vi "JSON Add Indent.vi"(8 "error in (no error)":errorcluster, 10 "Indent Size (2)":u32=2, 11 "JSON String":string) -> (0 "error out":errorcluster, 3 "Indented JSON String":string)   [LabVIEW 2020, in "RxnRover.lvlib" / "File IO.lvlib" / "JSON Utilities.lvlib"]
doc: "Adds indentation to the JSON string provided. The string must already have newlines added for indentation to be useful."
uses:
  JSON Utilities.lvlib
  <vilib>/regexp/Match Regular Expression.xnode
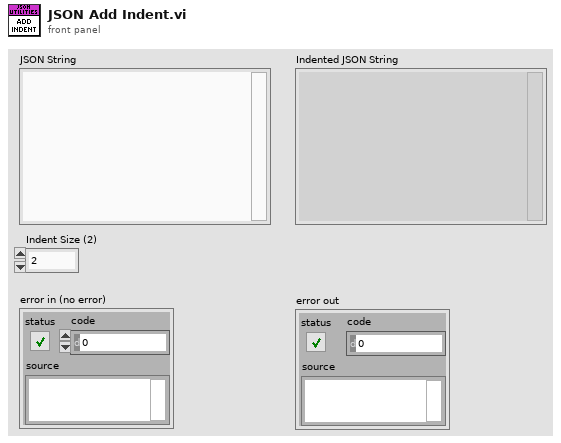
[diagram p1: front panel]
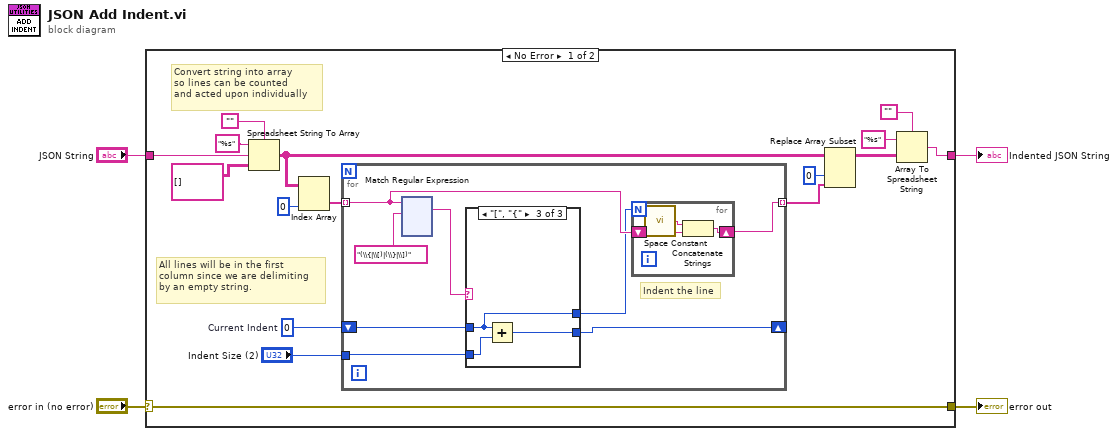
[diagram p0: block diagram]
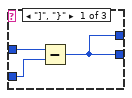
[diagram p2: hidden frame]
diagram:
  n1 = case shown="No Error" "error in (no error)" {
    selector: "error in (no error)" -> [w5 w154]
    tunnel: "JSON String" -> [w19 w153]
    tunnel: [w8 w153] -> w3
    tunnel: [w5 w154] -> w1
    frame No Error {
      w6 = 0  # Current Indent
      # "All lines will be in the first\ncolumn since we are delimiting\nby an empty string."
      # "Convert string into array\nso lines can be counted\nand acted upon individually"
      n2 = Spreadsheet String To Array(delimiter (Tab)="", format string="%s", spreadsheet string=w19, array type (2D Dbl)=string[][] []) -> (array=w16:string[][])
      n3 = Index Array(array=w16, index (col)=0 ("disabled index (col)")) -> (element=w17:string[])  [unwired: 1 in]
      n4 = for {
        tunnel: w17 -> [w24] mode=indexing
        tunnel: [w23] -> w14 mode=indexing
        tunnel: "Indent Size (2)" -> [w26]
        shift-right: [w22] -> _
        shift-left: w6 -> [w27]
        # "Indent the line"
        n5 = xnode "Match Regular Expression"("input string"=w24, "regular expression"="(\\{|\\[)|(\\}|\\])") -> ("whole match"=w25:string)  [unwired: 4 in, 4 out]
        n6 = case shown="\"[\", \"{\"" w25 {
          tunnel: w27 -> [w34 w35 w36]
          tunnel: w26 -> [w33 _ w38]
          tunnel: [w32 w35 w37] -> w22
          tunnel: [w32 w35 w36] -> w21
          frame "]", "}" {
            n7 = Subtract(x=w34, y=w33) -> (x-y=w32:u32)
          }
          frame Default {
          }
          frame "[", "{" {
            n8 = Add(x=w36, y=w38) -> (x+y=w37:u32)
          }
        }
        n9 = for {
          N: w21 -> [_]
          shift-right: [w29] -> w23
          shift-left: w24 -> [w31]
          n10 = call <vilib>:"Space Constant.vi"() -> ("String"=w30:string)
          n11 = Concatenate Strings(w30, w31) -> (w29:string)
        }
      }
      n12 = Replace Array Subset(array=w16, new element=w14, index (col)=0 ("disabled index (col)")) -> (w13:string[][])  [unwired: 1 in]
      n13 = Array To Spreadsheet String(delimiter (Tab)="", array=w13, 3:"%s") -> (spreadsheet string=w8:string)
    }
    frame Error {
    }
  }
  "Indented JSON String" <- w3
  "error out" <- w1
